vi "Execute.vi"(8 "error in (no error)":errorcluster, 11 "File Reader in":refnum<class "File Reader.lvclass">) -> (0 "error out":errorcluster, 2 "Data":dbl[](array[numeric]), 3 "File Reader out":refnum<class "File Reader.lvclass">)   [LabVIEW 2021, in "File Reader.lvclass"]
uses:
  File Reader.lvclass
  File Reader.lvclass/File Reader.ctl
  <vilib>/Utility/file.llb/Read Delimited Spreadsheet (DBL).vi
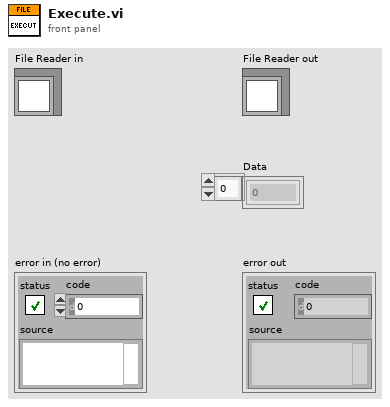
[diagram p1: front panel]
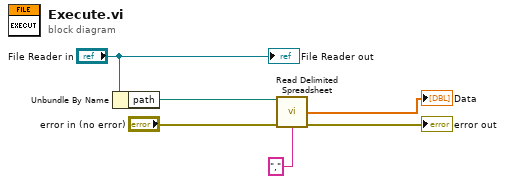
[diagram p0: block diagram]
diagram:
  n1 = Unbundle By Name("File Reader in") -> ("path"=w1:path)
  n2 = call-poly <vilib>:"Read Delimited Spreadsheet.vi"("file path (dialog if empty)"=w1, "error in (no error)"="error in (no error)", "delimiter (\\t)"="," ("delimiter (\\t)")) -> ("first row"=→"Data":dbl[], "error out"=→"error out":errorcluster)  [unwired: 7 in, 4 out]
  "File Reader out" <- "File Reader in"
